vi "ReadFileData.vi"(2 "RF lines":u32, 3 "Correct Delay?":bool=TRUE, 4 "RF Points":u32, 5 "Delay mics":sgl format="%_6g", 6 "yee delay":sgl, 7 "File Path":path) -> (1 "Data":i16[][](array[numeric]))   [LabVIEW 2022 SP3]
panel:
  in  "Reverse?":bool
  out "Data Points":u32
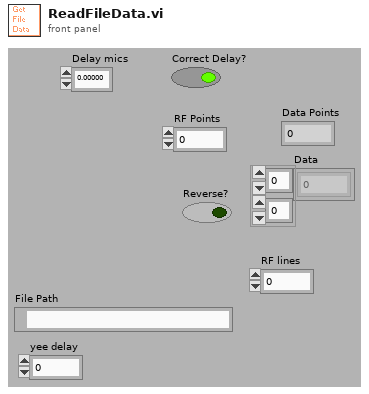
[diagram p1: front panel]
types:
  T1 = enum16{"big-endian, network order", "native, host order", "little-endian"}
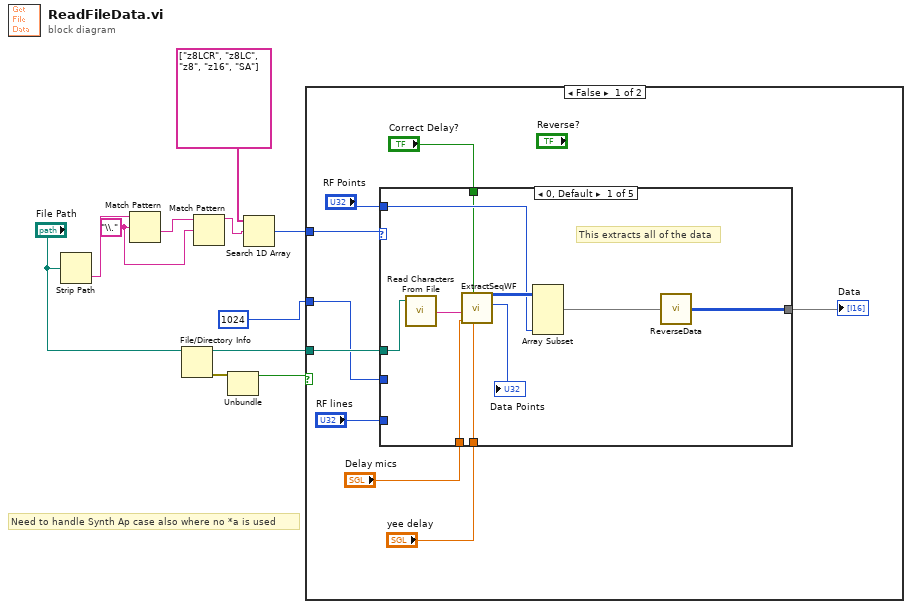
[diagram p0: block diagram]
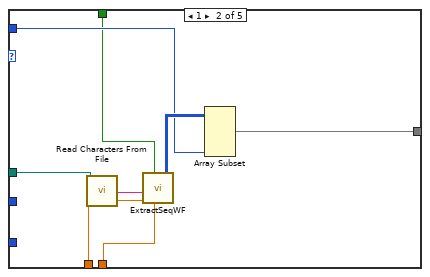
[diagram p2: hidden frame]
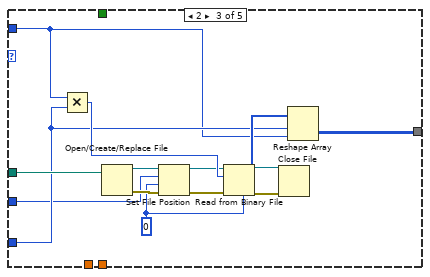
[diagram p3: hidden frame]
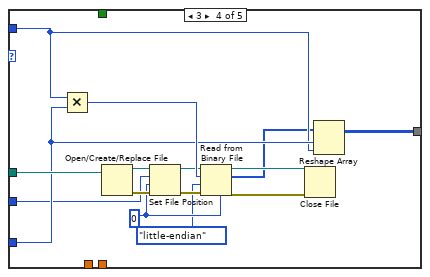
[diagram p4: hidden frame]
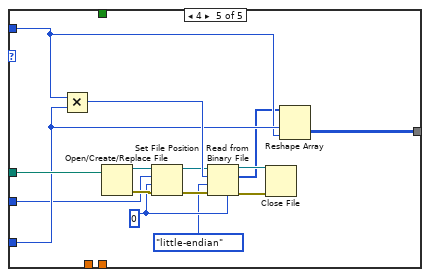
[diagram p5: hidden frame]
diagram:
  w8 = "\\."
  # "Need to handle Synth Ap case also where no *a is used"
  n1 = Strip Path(path="File Path") -> (name=w9:string)  [unwired: 1 out]
  n2 = Match Pattern(string=w9, regular expression=w8) -> (after substring=w7:string)  [unwired: 4 out]
  n3 = File/Directory Info(path="File Path") -> (path out=w2:path, error out=w4:errorcluster)  [unwired: 1 in, 5 out]
  n4 = Match Pattern(string=w7, regular expression=w8) -> (before substring=w6:string)  [unwired: 4 out]
  n5 = Unbundle(w4) -> ("status"=w3:bool)  [unwired: 2 out]
  n6 = Search 1D Array(1D array=string[] ["z8LCR", "z8LC", "z8", "z16", "SA"], element=w6) -> (index of element=w10:i32)  [unwired: 1 out]
  n7 = case shown="False" w3 {
    tunnel: w10 -> [w20 _]
    tunnel: w2 -> [w14 _]
    tunnel: 1024 -> [w13 _]
    frame False {
      n8 = case shown="0, Default" w20 {
        tunnel: "RF Points" -> [w27 w36 w45 w61 w76]
        tunnel: [w21 w31 w39 w55 w70] -> w19
        tunnel: "RF lines" -> [_ _ w46 w62 w77]
        tunnel: "Delay mics" -> [w26 w35 _ _ _]
        tunnel: "yee delay" -> [w25 w34 _ _ _]
        tunnel: w13 -> [_ _ w43 w59 w74]
        tunnel: w14 -> [w24 w33 w49 w64 w79]
        tunnel: "Correct Delay?" -> [w23 w32 _ _ _]
        frame 0, Default {
          # "This extracts all of the data"
          n9 = call <vilib>:"Read Characters From File.vi"("file path (dialog if empty)"=w24) -> ("character string"=w28:string)  [unwired: 1 in, 7 out]
          n10 = call "ExtractSeqWF.vi"("yee delay"=w25, "Correct Delay?"=w23, "Acqiris delay"=w26, "String"=w28) -> ("Data Pts"=→"Data Points":i32, "Data"=w30:i8[][])  [unwired: 2 in, 2 out]
          n11 = Array Subset(array=w30, length (col)=w27) -> (w22:i8[][])  [unwired: 3 in]
          n12 = call "ReverseData.vi"("Array in"=w22) -> ("Array out"=w21:i16[][])
        }
        frame 1 {
          n13 = call <vilib>:"Read Characters From File.vi"("file path (dialog if empty)"=w33) -> ("character string"=w37:string)  [unwired: 1 in, 7 out]
          n14 = call "ExtractSeqWF.vi"("yee delay"=w34, "Correct Delay?"=w32, "Acqiris delay"=w35, "String"=w37) -> ("Data"=w38:i8[][])  [unwired: 2 in, 3 out]
          n15 = Array Subset(array=w38, length (col)=w36) -> (w31:i8[][])  [unwired: 3 in]
        }
        frame 2 {
          w42 = i8 0
          n16 = Multiply(x=w45, y=w46) -> (x*y=w48:u32)
          n17 = Open/Create/Replace File(file path (use dialog)=w49) -> (refnum out=w50:refnum<file>, error out=w44:errorcluster)  [unwired: 1 in, 5 out]
          n18 = Set File Position(offset (in bytes) (0)=w43, refnum=w50, from (0:start)=w42, error in=w44) -> (refnum out=w41:refnum<file>, error out=w40:errorcluster)
          n19 = Read from Binary File(5:w42, 8:w40, 10:w48, 11:w41) -> (0:w51:errorcluster, 2:w47:i8[], 3:w52:refnum<file>)  [unwired: 3 out]
          n20 = Close File(refnum=w52, error in=w51) -> ()  [unwired: 2 out]
          n21 = Reshape Array(w47, w46, w45) -> (w39:i8[][])
        }
        frame 3 {
          w58 = i16 0
          n22 = Multiply(x=w61, y=w62) -> (x*y=w63:u32)
          n23 = Open/Create/Replace File(file path (use dialog)=w64) -> (refnum out=w65:refnum<file>, error out=w60:errorcluster)  [unwired: 1 in, 5 out]
          n24 = Set File Position(offset (in bytes) (0)=w59, refnum=w65, from (0:start)=w58, error in=w60) -> (refnum out=w57:refnum<file>, error out=w56:errorcluster)
          n25 = Read from Binary File(5:w58, 8:w56, 9:T1."little-endian" ("byte order (0:big-endian, network order)"), 10:w63, 11:w57) -> (0:w66:errorcluster, 2:w53:i16[], 3:w67:refnum<file>)  [unwired: 2 out]
          n26 = Close File(refnum=w67, error in=w66) -> ()  [unwired: 2 out]
          n27 = Reshape Array(w53, w62, w61) -> (w55:i16[][])
        }
        frame 4 {
          w73 = i16 0
          n28 = Multiply(x=w76, y=w77) -> (x*y=w78:u32)
          n29 = Open/Create/Replace File(file path (use dialog)=w79) -> (refnum out=w80:refnum<file>, error out=w75:errorcluster)  [unwired: 1 in, 5 out]
          n30 = Set File Position(offset (in bytes) (0)=w74, refnum=w80, from (0:start)=w73, error in=w75) -> (refnum out=w72:refnum<file>, error out=w71:errorcluster)
          n31 = Read from Binary File(5:w73, 8:w71, 9:T1."little-endian" ("byte order (0:big-endian, network order)"), 10:w78, 11:w72) -> (0:w81:errorcluster, 2:w68:i16[], 3:w82:refnum<file>)  [unwired: 2 out]
          n32 = Close File(refnum=w82, error in=w81) -> ()  [unwired: 2 out]
          n33 = Reshape Array(w68, w77, w76) -> (w70:i16[][])
        }
      }
      "Data" <- w19
    }
    frame True {
    }
  }
